vi "Graphe_XY.vi"(0 "Graphe":T1(graph), 3 "Tableau de chaînes":string[](array[string])) -> ()   [LabVIEW 2013]
uses:
  <vilib>/Utility/miscctls.llb/LVPositionTypeDef.ctl
  <vilib>/Utility/miscctls.llb/LVPointTypeDef.ctl
panel:
  in  "Bouton Aide":bool
  in  "Active maths":bool
  out "Nbre courbes":i32
  in  "Quitter graphe":bool
  in  "Palette:Outil actif":i32
  in  "Curseur visible":bool
  in  "Tout sélectionner":bool
  in  "Curseur":u16(ring)
  in  "Quadrillage":u16(ring)=1 items=["Sans", "Horizontal", "Vertical", "Tout"]
  in  "Mini":dbl max=19.999 format="%#.3f"
  in  "Maxi":dbl min=0.001 format="%#.3f"
  in  "Echelle Y":u16(ring) items=["Manu"=0, "Auto"=2]
  out "Y":dbl format="%#.3g"
  out "X":timestamp format="%<%X\n%x>T"
  out "residue 2":dbl caption="résidu"
  out "offset":dbl
  out "damping":dbl caption="atténuation"
  out "amplitude":dbl
  out "R-square":dbl caption="R carré"
  out "residue":dbl caption="résidu"
  out "intercept":dbl caption="interception"
  out "slope":dbl caption="pente"
  out "Intégrale":dbl format="%0.4f"
  out "variance":dbl format="%0.2f"
  out "standard deviation":dbl caption="écart-type" format="%0.2f"
  out "valeur max":dbl
  out "valeur min":dbl
  out "mean":dbl caption="moyenne" format="%0.2f"
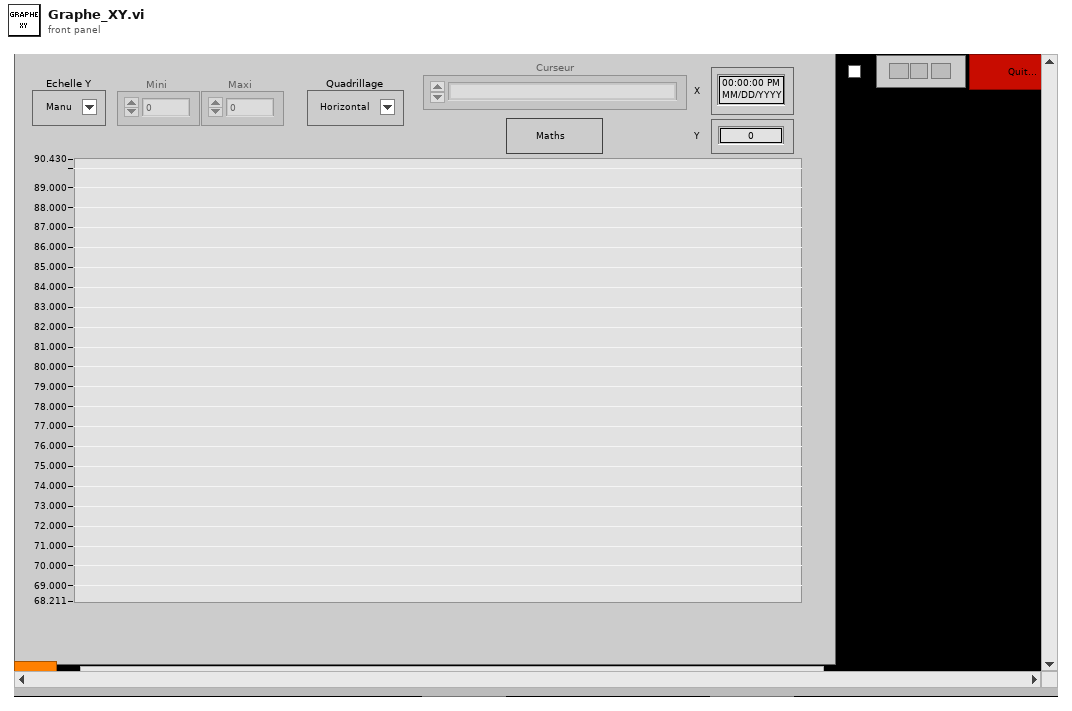
[diagram p1: front panel]
types:
  T1 = cluster{"Horodatage":timestamp[], "Donnees":dbl[]}[]
  T2 = typedef "LVPositionTypeDef.ctl" = cluster{"Left":i32, "Top":i32}
  T3 = typedef "LVPointTypeDef.ctl" = cluster{"Horizontal":i16, "Vertical":i16}
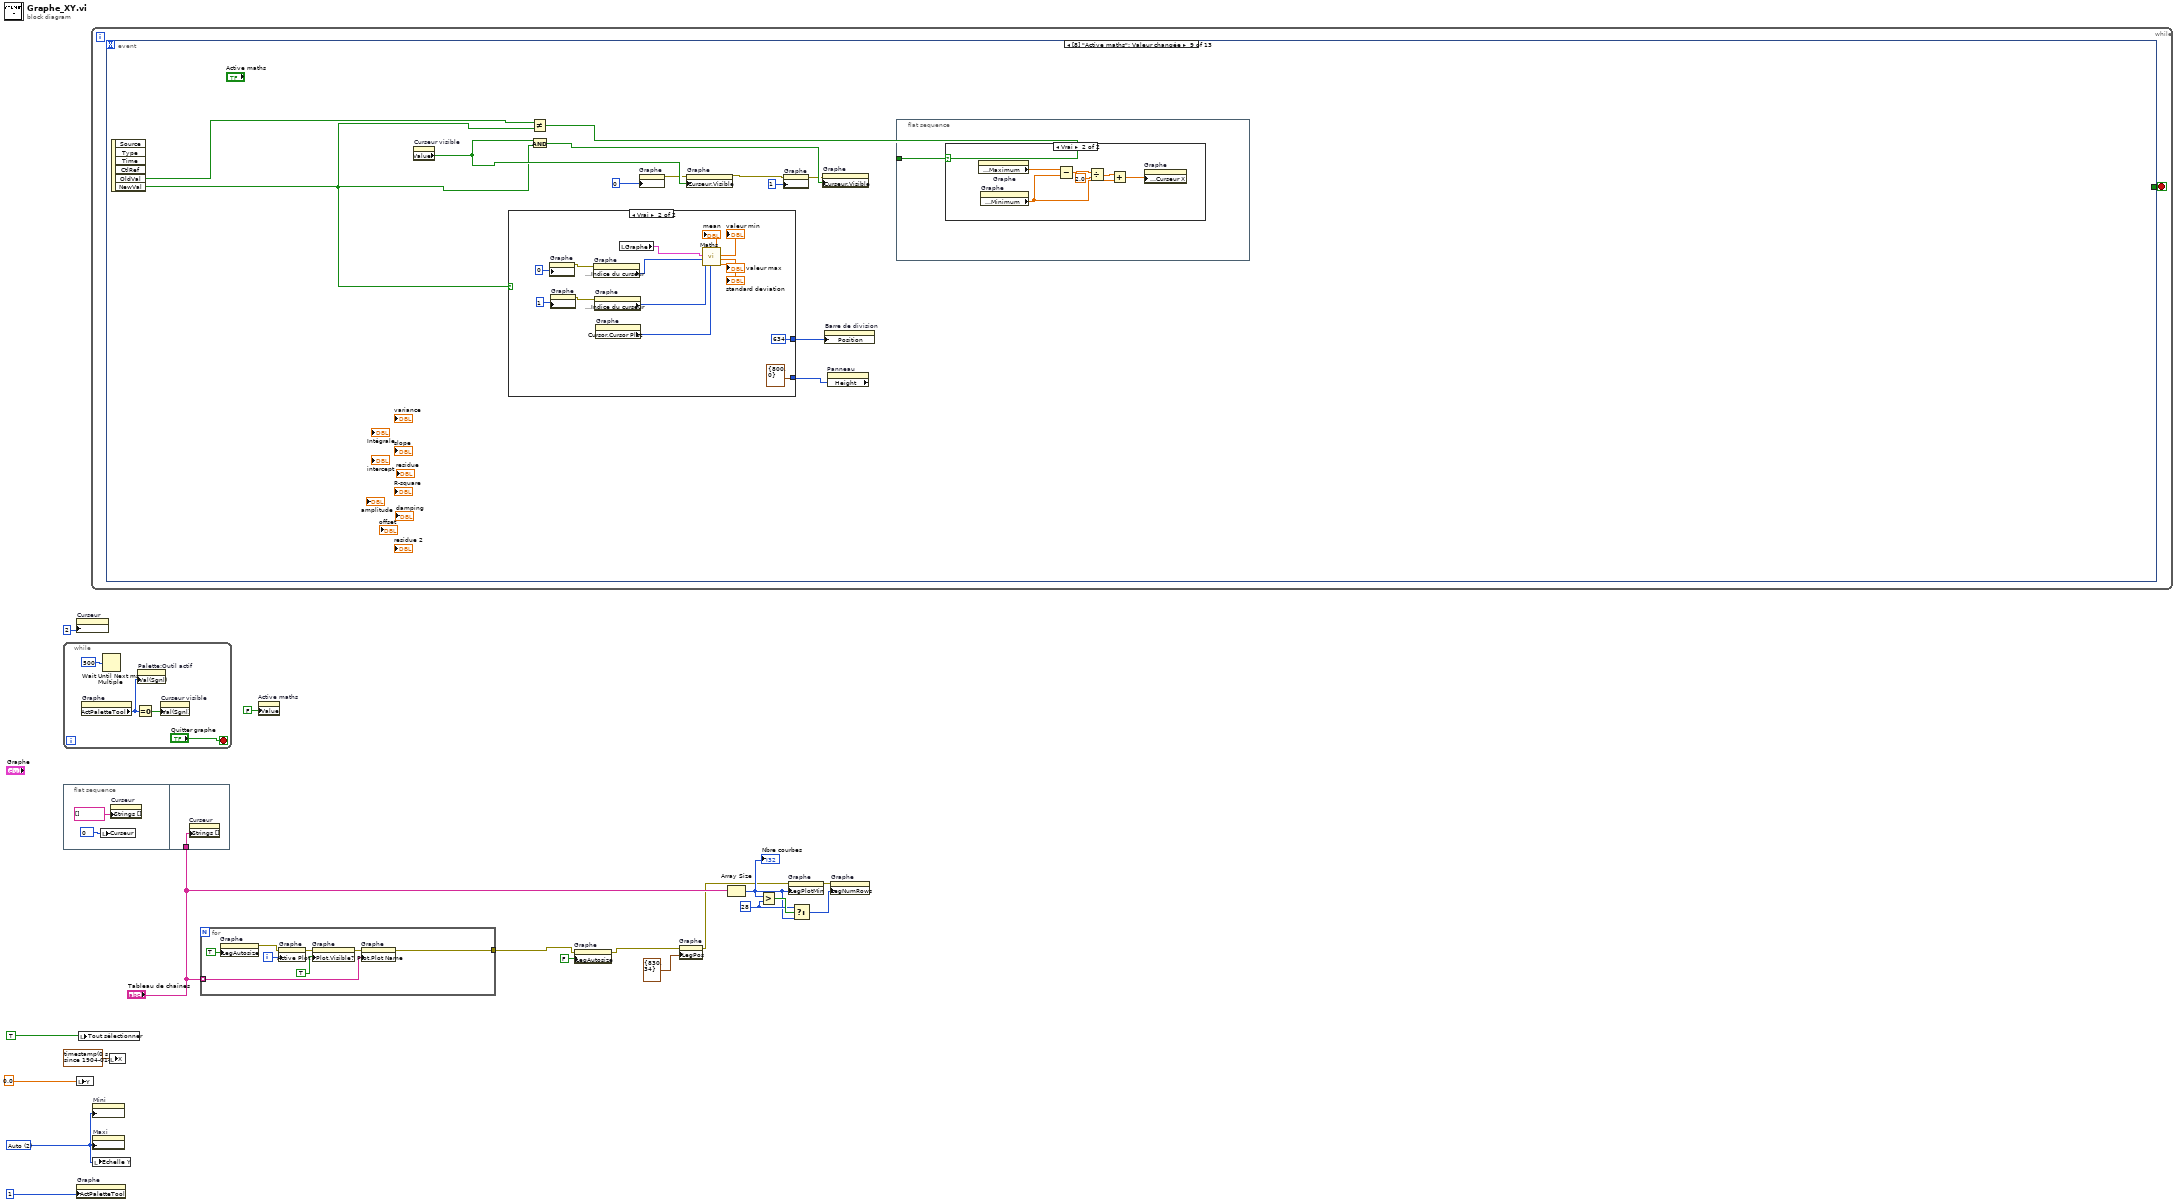
[diagram p0: block diagram]
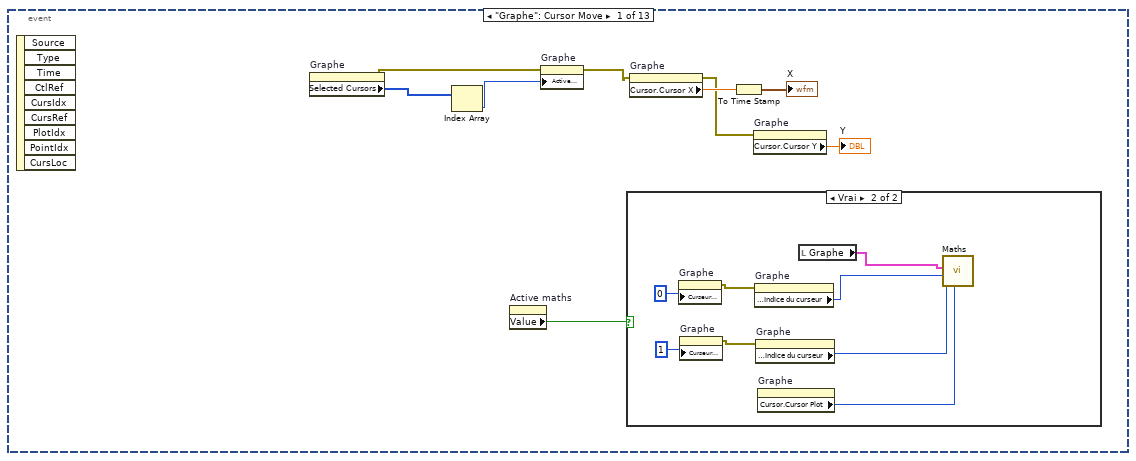
[diagram p2: hidden frame]
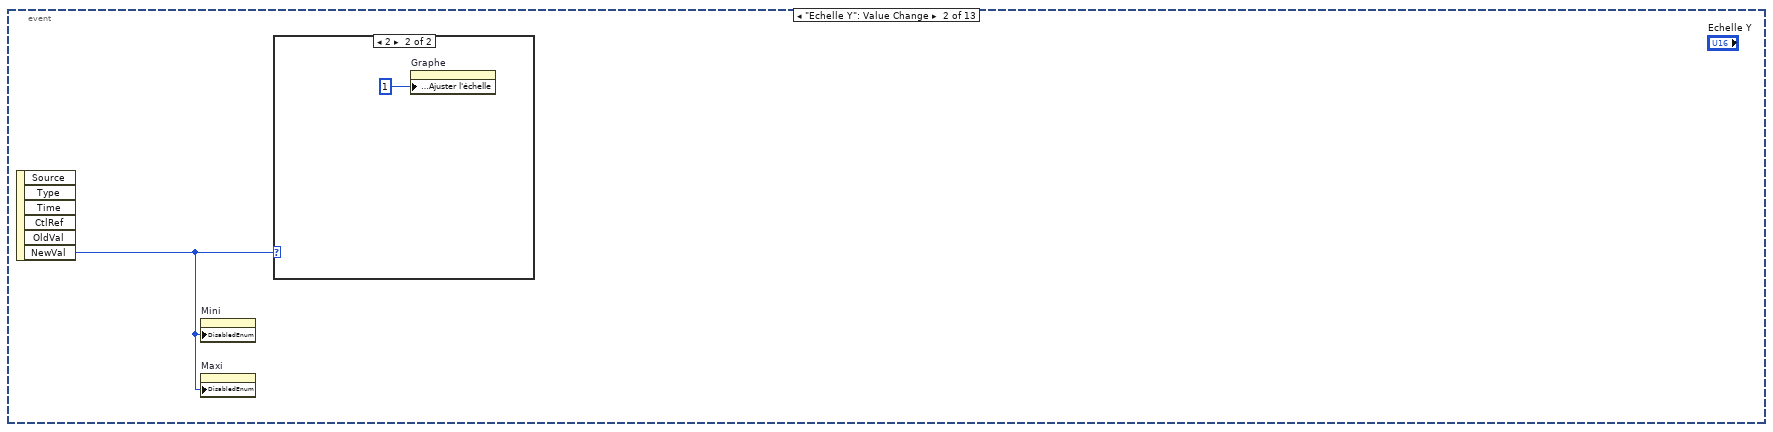
[diagram p4: hidden frame]
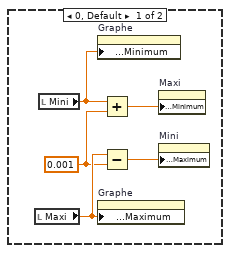
[diagram p5: hidden frame]
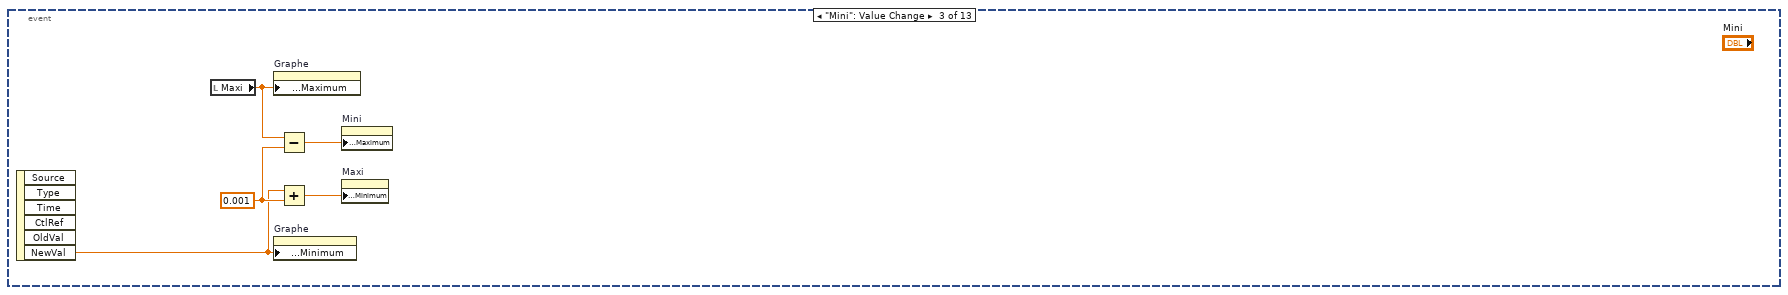
[diagram p6: hidden frame]
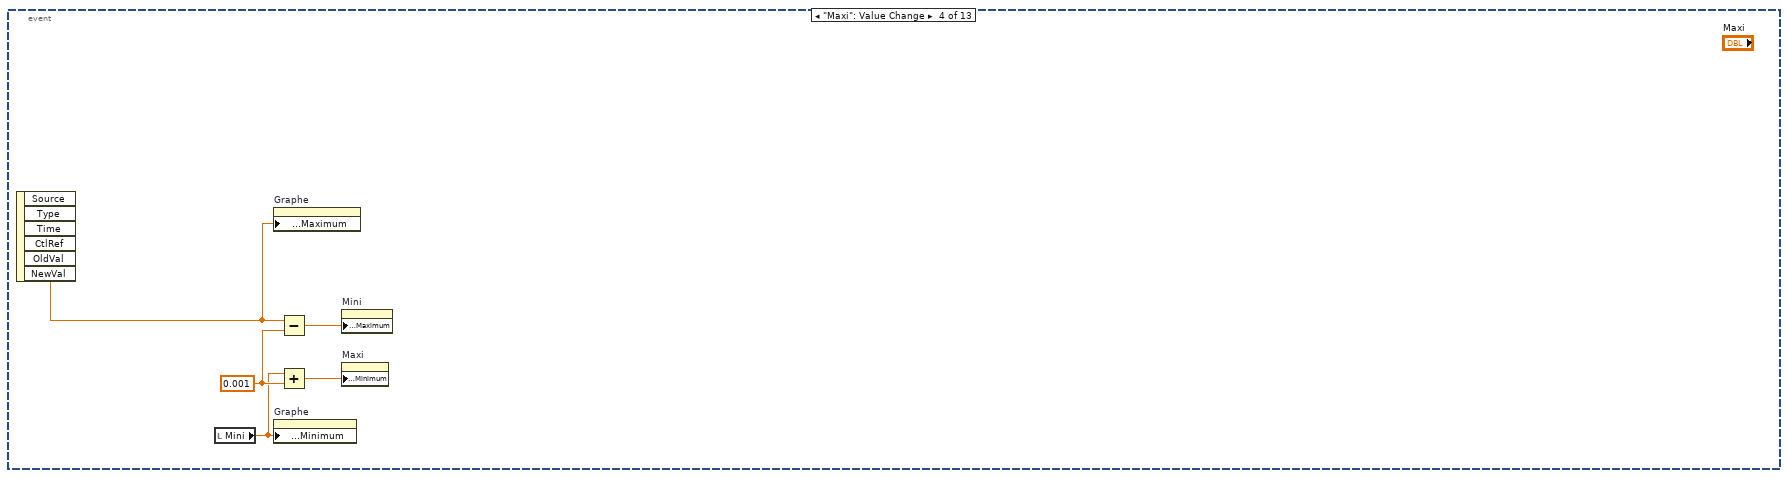
[diagram p7: hidden frame]
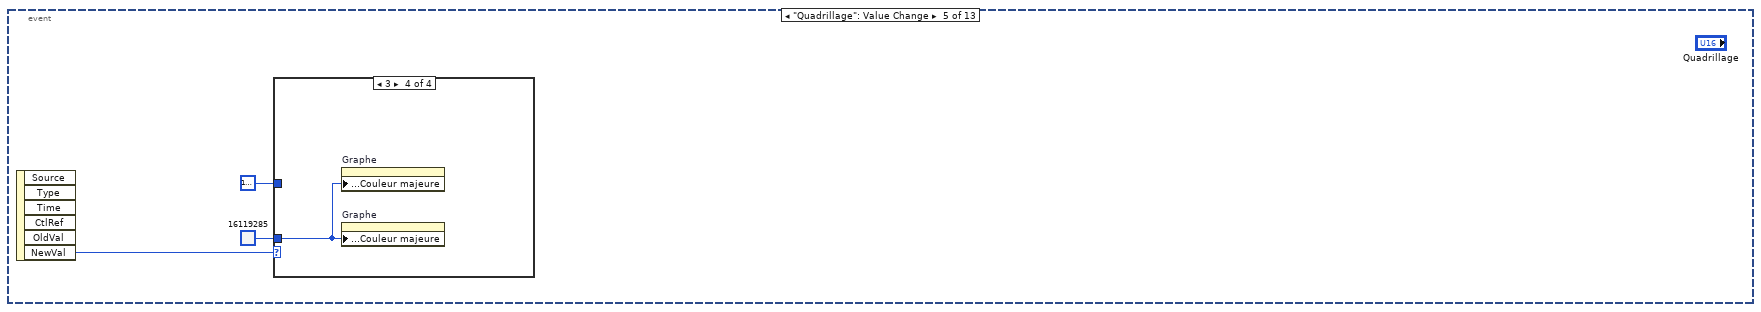
[diagram p8: hidden frame]
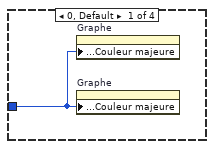
[diagram p9: hidden frame]
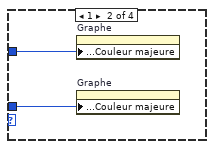
[diagram p10: hidden frame]
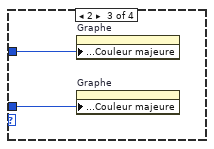
[diagram p11: hidden frame]
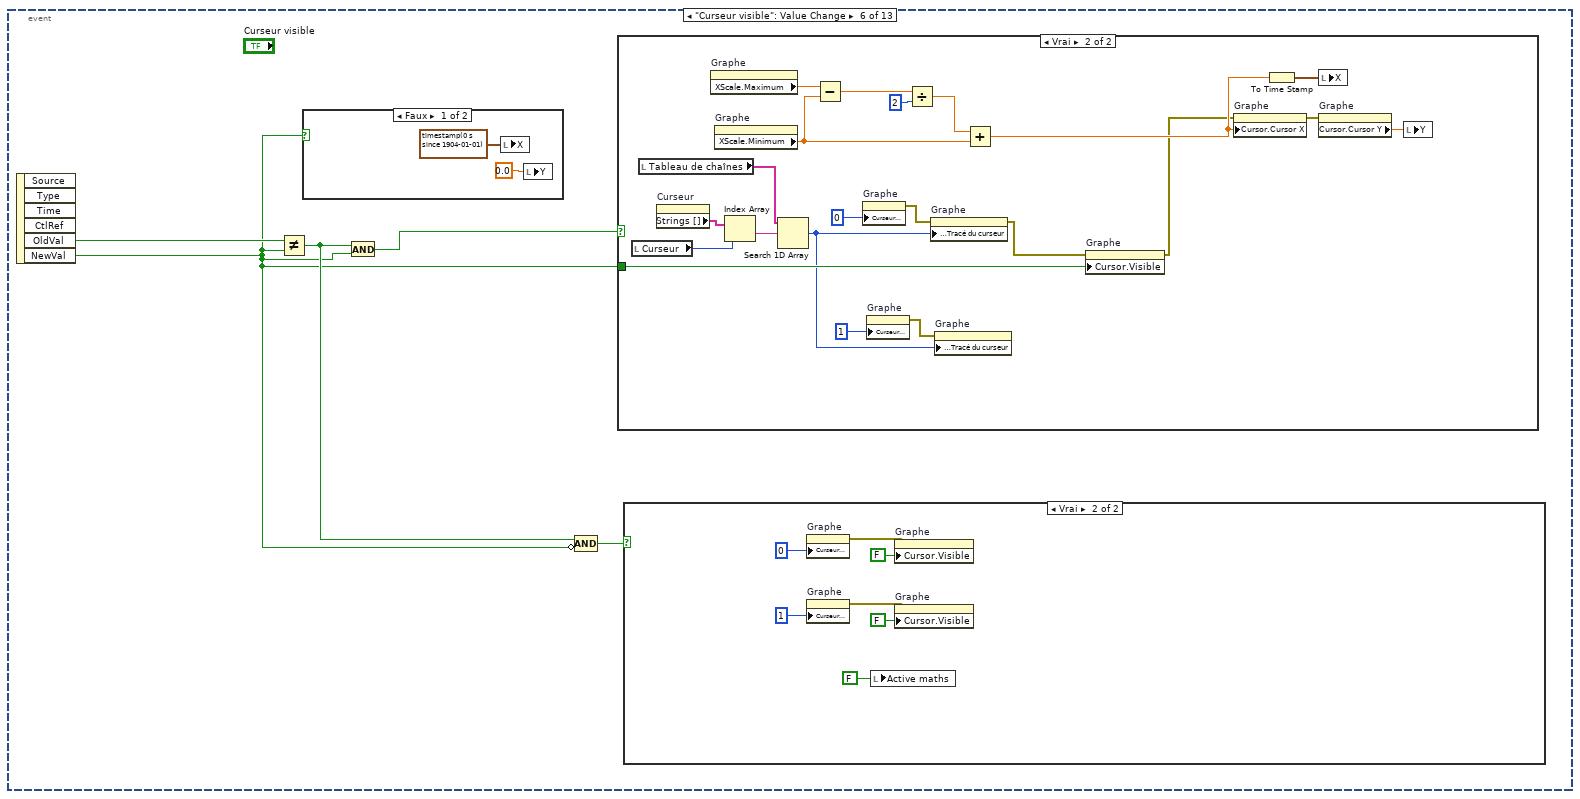
[diagram p12: hidden frame]
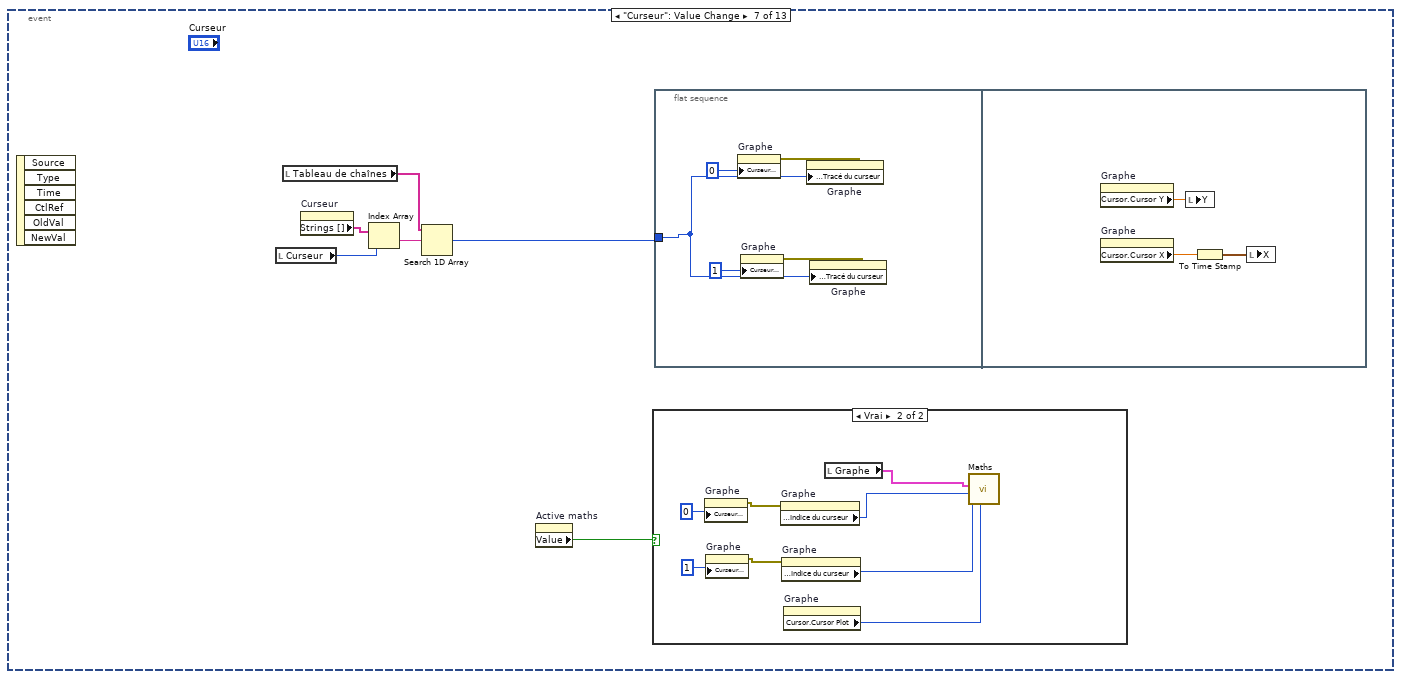
[diagram p16: hidden frame]
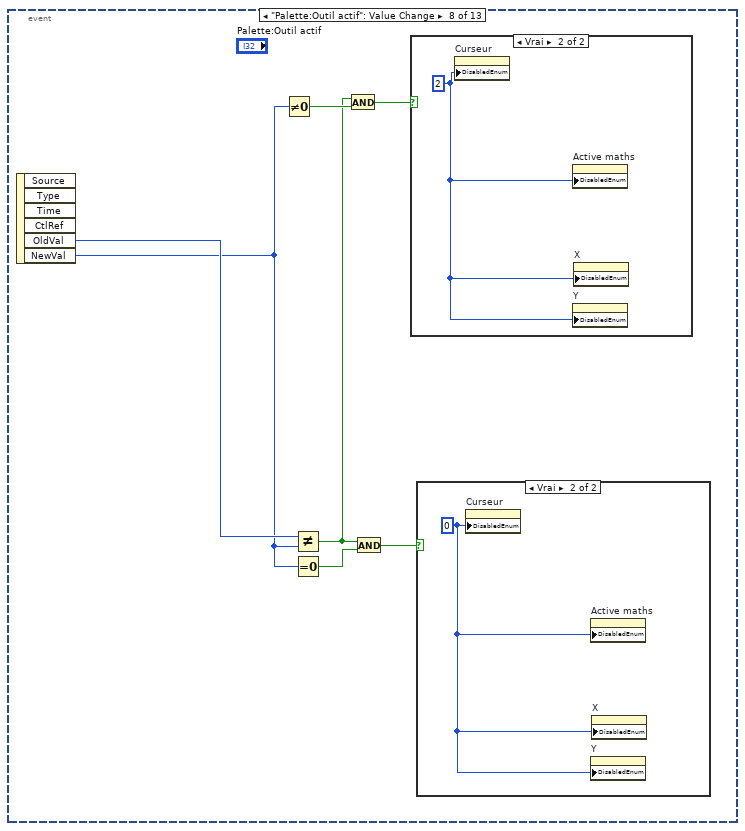
[diagram p18: hidden frame]
diagram:
  w9 = 28 ("y")
  w18 = u16 2 items=["Manu"=0, "Auto"=2] ("Echelle Y")
  n1 = while {
    stop <- "Quitter graphe" stop-if-true
    n2 = property on="Graphe" class="GraphXY (strict)"() -> ("ActPaletteTool"=w20:i32)  [unwired: 2 in, 2 out]
    n3 = Wait Until Next ms Multiple(millisecond multiple=u32 500 ("n millisecondes")) -> ()  [unwired: 1 out]
    n4 = Equal To 0?(x=w20) -> (x = 0?=w21:bool)
    n5 = property on="Palette:Outil actif" class="NumNb (strict)"("Val(Sgnl)"=w20) -> ()  [unwired: 2 in, 2 out]
    n6 = property on="Curseur visible" class="Bool (strict)"("Val(Sgnl)"=w21) -> ()  [unwired: 2 in, 2 out]
  }
  n7 = flat-sequence {
    tunnel: "Tableau de chaînes" -> [w25]
    frame #0 {
      w24 = u16 0 items=[""] ("Curseur")
      n8 = local write "Curseur"(w24) -> ()
      n9 = property on="Curseur" class="MDér (strict)"("Strings []"=string[] [] ("Chaînes []")) -> ()  [unwired: 2 in, 2 out]
    }
    frame #1 {
      n10 = property on="Curseur" class="MDér (strict)"("Strings []"=w25) -> ()  [unwired: 2 in, 2 out]
    }
  }
  n11 = property on="Curseur" class="MDér (strict)"("DisabledEnum"=i8 2 ("cas vrai")) -> ()  [unwired: 2 in, 2 out]
  n12 = local write "Y"(0.0 ("Y")) -> ()
  n13 = property on="Graphe" class="GraphXY (strict)"("ActPaletteTool"=1 ("Palette:Outil actif")) -> ()  [unwired: 2 in, 2 out]
  n14 = local write "Tout sélectionner"(TRUE ("Tout sélectionner")) -> ()
  n15 = while {
    stop <- w26 stop-if-true
    n16 = event shown="[8] \"Active maths\": Valeur changée" {
      selector: _ -> [_ _ _ _ _ _ _ _ _ _ _ _ _]
      dyn-events: _ -> [_ _ _ _ _ _ _ _ _ _ _ _ _]
      timeout: _ -> [_ _ _ _ _ _ _ _ _ _ _ _ _]
      tunnel: [_ _ _ _ _ _ _ _ _ _ _ w241 _] -> w26
      event "Graphe": Cursor Move {
        n17 = event-data() -> ()  [unwired: 1 in, 9 out]
        n18 = property on="Graphe" class="GraphXY (strict)"() -> (error out=w29:errorcluster, "Selected Cursors"=w31:u32[])  [unwired: 2 in, 1 out]
        n19 = Index Array(array=w31) -> (element=w30:u32)  [unwired: 1 in]
        n20 = property on="Active maths" class="Bool (strict)"() -> ("Value"=w27:bool)  [unwired: 2 in, 2 out]
        n21 = property on="Graphe" class="GraphXY (strict)"(error in=w29, "Active Cursor"=w30) -> (error out=w28:errorcluster)  [unwired: 1 in, 1 out]
        n22 = case shown="Vrai" w27 {
          frame False {
          }
          frame True {
            n23 = property on="Graphe" class="GraphXY (strict)"("Curseur actif"=u32 0) -> (error out=w43:errorcluster)  [unwired: 2 in, 1 out]
            n24 = property on="Graphe" class="GraphXY (strict)"("Curseur actif"=u32 1) -> (error out=w39:errorcluster)  [unwired: 2 in, 1 out]
            n25 = property on="Graphe" class="GraphXY (strict)"(error in=w43) -> ("Curseur.Indice du curseur"=w41:i32)  [unwired: 1 in, 2 out]
            n26 = property on="Graphe" class="GraphXY (strict)"(error in=w39) -> ("Curseur.Indice du curseur"=w38:i32)  [unwired: 1 in, 2 out]
            n27 = property on="Graphe" class="GraphXY (strict)"() -> ("Cursor.Cursor Plot"=w37:i32)  [unwired: 2 in, 2 out]
            n28 = local read "Graphe"() -> (w36:T1)
            n29 = call "Maths.vi"("Curseur tracé"=w37, "Indice curseur 2"=w38, "Indice curseur 1"=w41, "Graphe"=w36) -> ()  [unwired: 4 in, 4 out]
          }
        }
        n30 = property on="Graphe" class="GraphXY (strict)"(error in=w28) -> (error out=w32:errorcluster, "Cursor.Cursor X"=w34:dbl)  [unwired: 1 in, 1 out]
        n31 = To Time Stamp(1:w34) -> (0:→"X":timestamp)
        n32 = property on="Graphe" class="GraphXY (strict)"(error in=w32) -> ("Cursor.Cursor Y"=→"Y":dbl)  [unwired: 1 in, 2 out]
      }
      event "Echelle Y": Value Change {
        n33 = event-data() -> ("NewVal"=w44:u16)  [unwired: 1 in, 5 out]
        n34 = property on="Mini" class="NumNb (strict)"("DisabledEnum"=w44) -> ()  [unwired: 2 in, 2 out]
        n35 = property on="Maxi" class="NumNb (strict)"("DisabledEnum"=w44) -> ()  [unwired: 2 in, 2 out]
        n36 = case shown="2" w44 {
          frame 0, Default {
            w48 = 0.001 ("y")
            n37 = local read "Maxi"() -> (w49:dbl)
            n38 = local read "Mini"() -> (w45:dbl)
            n39 = property on="Graphe" class="GraphXY (strict)"("Échelle des Y.Gamme:Minimum"=w45) -> ()  [unwired: 2 in, 2 out]
            n40 = property on="Graphe" class="GraphXY (strict)"("Échelle des Y.Gamme:Maximum"=w49) -> ()  [unwired: 2 in, 2 out]
            n41 = Add(x=w45, y=w48) -> (x+y=w46:dbl)
            n42 = Subtract(x=w49, y=w48) -> (x-y=w47:dbl)
            n43 = property on="Maxi" class="NumNb (strict)"("Limites d'entrée des données:Minimum"=w46) -> ()  [unwired: 2 in, 2 out]
            n44 = property on="Mini" class="NumNb (strict)"("Limites d'entrée des données:Maximum"=w47) -> ()  [unwired: 2 in, 2 out]
          }
          frame 2 {
            n45 = property on="Graphe" class="GraphXY (strict)"("Échelle des Y.Ajuster l'échelle"=u8 1 ("Échelle Y.Ajuster l'échelle")) -> ()  [unwired: 2 in, 2 out]
          }
        }
      }
      event "Mini": Value Change {
        w54 = 0.001 ("y")
        n46 = event-data() -> ("NewVal"=w51:dbl)  [unwired: 1 in, 5 out]
        n47 = local read "Maxi"() -> (w55:dbl)
        n48 = property on="Graphe" class="GraphXY (strict)"("Échelle des Y.Gamme:Maximum"=w55) -> ()  [unwired: 2 in, 2 out]
        n49 = property on="Graphe" class="GraphXY (strict)"("Échelle des Y.Gamme:Minimum"=w51) -> ()  [unwired: 2 in, 2 out]
        n50 = Subtract(x=w55, y=w54) -> (x-y=w53:dbl)
        n51 = Add(x=w51, y=w54) -> (x+y=w52:dbl)
        n52 = property on="Mini" class="NumNb (strict)"("Limites d'entrée des données:Maximum"=w53) -> ()  [unwired: 2 in, 2 out]
        n53 = property on="Maxi" class="NumNb (strict)"("Limites d'entrée des données:Minimum"=w52) -> ()  [unwired: 2 in, 2 out]
      }
      event "Maxi": Value Change {
        w60 = 0.001 ("y")
        n54 = event-data() -> ("NewVal"=w57:dbl)  [unwired: 1 in, 5 out]
        n55 = local read "Mini"() -> (w56:dbl)
        n56 = property on="Graphe" class="GraphXY (strict)"("Échelle des Y.Gamme:Maximum"=w57) -> ()  [unwired: 2 in, 2 out]
        n57 = property on="Graphe" class="GraphXY (strict)"("Échelle des Y.Gamme:Minimum"=w56) -> ()  [unwired: 2 in, 2 out]
        n58 = Subtract(x=w57, y=w60) -> (x-y=w59:dbl)
        n59 = Add(x=w56, y=w60) -> (x+y=w58:dbl)
        n60 = property on="Mini" class="NumNb (strict)"("Limites d'entrée des données:Maximum"=w59) -> ()  [unwired: 2 in, 2 out]
        n61 = property on="Maxi" class="NumNb (strict)"("Limites d'entrée des données:Minimum"=w58) -> ()  [unwired: 2 in, 2 out]
      }
      event "Quadrillage": Value Change {
        n62 = event-data() -> ("NewVal"=w63:u16)  [unwired: 1 in, 5 out]
        n63 = case shown="3" w63 {
          tunnel: u32 16119285 -> [_ w66 w68 w69]
          tunnel: u32 16777216 -> [w64 w65 w67 _]
          frame 0, Default {
            n64 = property on="Graphe" class="GraphXY (strict)"("Échelle des X.Couleurs de grille:Couleur majeure"=w64) -> ()  [unwired: 2 in, 2 out]
            n65 = property on="Graphe" class="GraphXY (strict)"("Échelle des Y.Couleurs de grille:Couleur majeure"=w64) -> ()  [unwired: 2 in, 2 out]
          }
          frame 1 {
            n66 = property on="Graphe" class="GraphXY (strict)"("Échelle des X.Couleurs de grille:Couleur majeure"=w65) -> ()  [unwired: 2 in, 2 out]
            n67 = property on="Graphe" class="GraphXY (strict)"("Échelle des Y.Couleurs de grille:Couleur majeure"=w66) -> ()  [unwired: 2 in, 2 out]
          }
          frame 2 {
            n68 = property on="Graphe" class="GraphXY (strict)"("Échelle des Y.Couleurs de grille:Couleur majeure"=w67) -> ()  [unwired: 2 in, 2 out]
            n69 = property on="Graphe" class="GraphXY (strict)"("Échelle des X.Couleurs de grille:Couleur majeure"=w68) -> ()  [unwired: 2 in, 2 out]
          }
          frame 3 {
            n70 = property on="Graphe" class="GraphXY (strict)"("Échelle des X.Couleurs de grille:Couleur majeure"=w69) -> ()  [unwired: 2 in, 2 out]
            n71 = property on="Graphe" class="GraphXY (strict)"("Échelle des Y.Couleurs de grille:Couleur majeure"=w69) -> ()  [unwired: 2 in, 2 out]
          }
        }
      }
      event "Curseur visible": Value Change {
        n72 = event-data() -> ("OldVal"=w74:bool, "NewVal"=w70:bool)  [unwired: 1 in, 4 out]
        n73 = Not Equal?(x=w74, y=w70) -> (x != y?=w72:bool)
        n74 = case shown="Faux" w70 {
          frame False {
            n75 = local write "X"(timestamp(0 s since 1904-01-01) ("X")) -> ()
            n76 = local write "Y"(0.0 ("Y")) -> ()
          }
          frame True {
          }
        }
        n77 = And(x=w72, y=w70) -> (x .and. y?=w73:bool)
        n78 = Compound Arithmetic op=AND(w72, invert w70) -> (w71:bool)
        n79 = case shown="Vrai" w73 {
          tunnel: w70 -> [_ w94]
          frame False {
          }
          frame True {
            n80 = local read "Curseur"() -> (w89:u16)
            n81 = local read "Tableau de chaînes"() -> (w92:string[])
            n82 = property on="Curseur" class="MDér (strict)"() -> ("Strings []"=w90:string[])  [unwired: 2 in, 2 out]
            n83 = property on="Graphe" class="GraphXY (strict)"() -> ("XScale.Maximum"=w103:dbl)  [unwired: 2 in, 2 out]
            n84 = property on="Graphe" class="GraphXY (strict)"() -> ("XScale.Minimum"=w100:dbl)  [unwired: 2 in, 2 out]
            n85 = Index Array(array=w90, index=w89) -> (element=w91:string)
            n86 = Search 1D Array(1D array=w92, element=w91) -> (index of element=w86:i32)  [unwired: 1 in]
            n87 = Subtract(x=w103, y=w100) -> (x-y=w102:dbl)
            n88 = property on="Graphe" class="GraphXY (strict)"("Curseur actif"=u32 0) -> (error out=w93:errorcluster)  [unwired: 2 in, 1 out]
            n89 = property on="Graphe" class="GraphXY (strict)"("Curseur actif"=u32 1) -> (error out=w88:errorcluster)  [unwired: 2 in, 1 out]
            n90 = Divide(x=w102, y=2) -> (x/y=w101:dbl)
            n91 = property on="Graphe" class="GraphXY (strict)"(error in=w93, "Curseur.Tracé du curseur"=w86) -> (error out=w84:errorcluster)  [unwired: 1 in, 1 out]
            n92 = property on="Graphe" class="GraphXY (strict)"(error in=w88, "Curseur.Tracé du curseur"=w86) -> ()  [unwired: 1 in, 2 out]
            n93 = Add(x=w101, y=w100) -> (x+y=w97:dbl)
            n94 = property on="Graphe" class="GraphXY (strict)"(error in=w84, "Cursor.Visible"=w94) -> (error out=w85:errorcluster)  [unwired: 1 in, 1 out]
            n95 = property on="Graphe" class="GraphXY (strict)"(error in=w85, "Cursor.Cursor X"=w97) -> (error out=w96:errorcluster)  [unwired: 1 in, 1 out]
            n96 = To Time Stamp(1:w97) -> (0:w98:timestamp)
            n97 = local write "X"(w98) -> ()
            n98 = property on="Graphe" class="GraphXY (strict)"(error in=w96) -> ("Cursor.Cursor Y"=w99:dbl)  [unwired: 1 in, 2 out]
            n99 = local write "Y"(w99) -> ()
          }
        }
        n100 = case shown="Vrai" w71 {
          frame False {
          }
          frame True {
            n101 = property on="Graphe" class="GraphXY (strict)"("Curseur actif"=u32 0) -> (error out=w80:errorcluster)  [unwired: 2 in, 1 out]
            n102 = property on="Graphe" class="GraphXY (strict)"("Curseur actif"=u32 1) -> (error out=w77:errorcluster)  [unwired: 2 in, 1 out]
            n103 = local write "Active maths"(FALSE ("Selection math")) -> ()
            n104 = property on="Graphe" class="GraphXY (strict)"(error in=w80, "Cursor.Visible"=FALSE ("Curseur.Visible")) -> ()  [unwired: 1 in, 2 out]
            n105 = property on="Graphe" class="GraphXY (strict)"(error in=w77, "Cursor.Visible"=FALSE ("Curseur.Visible")) -> ()  [unwired: 1 in, 2 out]
          }
        }
      }
      event "Curseur": Value Change {
        n106 = event-data() -> ()  [unwired: 1 in, 6 out]
        n107 = local read "Curseur"() -> (w106:u16)
        n108 = local read "Tableau de chaînes"() -> (w109:string[])
        n109 = property on="Curseur" class="MDér (strict)"() -> ("Strings []"=w107:string[])  [unwired: 2 in, 2 out]
        n110 = Index Array(array=w107, index=w106) -> (element=w108:string)
        n111 = Search 1D Array(1D array=w109, element=w108) -> (index of element=w105:i32)  [unwired: 1 in]
        n112 = property on="Active maths" class="Bool (strict)"() -> ("Value"=w110:bool)  [unwired: 2 in, 2 out]
        n113 = case shown="Vrai" w110 {
          frame False {
          }
          frame True {
            n114 = property on="Graphe" class="GraphXY (strict)"("Curseur actif"=u32 0) -> (error out=w118:errorcluster)  [unwired: 2 in, 1 out]
            n115 = property on="Graphe" class="GraphXY (strict)"("Curseur actif"=u32 1) -> (error out=w114:errorcluster)  [unwired: 2 in, 1 out]
            n116 = property on="Graphe" class="GraphXY (strict)"(error in=w118) -> ("Curseur.Indice du curseur"=w116:i32)  [unwired: 1 in, 2 out]
            n117 = property on="Graphe" class="GraphXY (strict)"(error in=w114) -> ("Curseur.Indice du curseur"=w113:i32)  [unwired: 1 in, 2 out]
            n118 = property on="Graphe" class="GraphXY (strict)"() -> ("Cursor.Cursor Plot"=w112:i32)  [unwired: 2 in, 2 out]
            n119 = local read "Graphe"() -> (w111:T1)
            n120 = call "Maths.vi"("Curseur tracé"=w112, "Indice curseur 2"=w113, "Indice curseur 1"=w116, "Graphe"=w111) -> ()  [unwired: 4 in, 4 out]
          }
        }
        n121 = flat-sequence {
          tunnel: w105 -> [w119]
          frame #0 {
            n122 = property on="Graphe" class="GraphXY (strict)"("Curseur actif"=u32 0) -> (error out=w122:errorcluster)  [unwired: 2 in, 1 out]
            n123 = property on="Graphe" class="GraphXY (strict)"("Curseur actif"=u32 1) -> (error out=w121:errorcluster)  [unwired: 2 in, 1 out]
            n124 = property on="Graphe" class="GraphXY (strict)"(error in=w122, "Curseur.Tracé du curseur"=w119) -> ()  [unwired: 1 in, 2 out]
            n125 = property on="Graphe" class="GraphXY (strict)"(error in=w121, "Curseur.Tracé du curseur"=w119) -> ()  [unwired: 1 in, 2 out]
          }
          frame #1 {
            n126 = property on="Graphe" class="GraphXY (strict)"() -> ("Cursor.Cursor Y"=w126:dbl)  [unwired: 2 in, 2 out]
            n127 = property on="Graphe" class="GraphXY (strict)"() -> ("Cursor.Cursor X"=w124:dbl)  [unwired: 2 in, 2 out]
            n128 = local write "Y"(w126) -> ()
            n129 = To Time Stamp(1:w124) -> (0:w125:timestamp)
            n130 = local write "X"(w125) -> ()
          }
        }
      }
      event "Palette:Outil actif": Value Change {
        n131 = event-data() -> ("OldVal"=w133:i32, "NewVal"=w129:i32)  [unwired: 1 in, 4 out]
        n132 = Not Equal To 0?(x=w129) -> (x != 0?=w130:bool)
        n133 = Not Equal?(x=w133, y=w129) -> (x != y?=w128:bool)
        n134 = Equal To 0?(x=w129) -> (x = 0?=w127:bool)
        n135 = And(x=w128, y=w130) -> (x .and. y?=w131:bool)
        n136 = And(x=w128, y=w127) -> (x .and. y?=w132:bool)
        n137 = case shown="Vrai" w131 {
          frame False {
          }
          frame True {
            w134 = i8 2 ("cas vrai")
            n138 = property on="Curseur" class="MDér (strict)"("DisabledEnum"=w134) -> ()  [unwired: 2 in, 2 out]
            n139 = property on="Active maths" class="Bool (strict)"("DisabledEnum"=w134) -> ()  [unwired: 2 in, 2 out]
            n140 = property on="Y" class="NumNb (strict)"("DisabledEnum"=w134) -> ()  [unwired: 2 in, 2 out]
            n141 = property on="X" class="TempsAbs (strict)"("DisabledEnum"=w134) -> ()  [unwired: 2 in, 2 out]
          }
        }
        n142 = case shown="Vrai" w132 {
          frame False {
          }
          frame True {
            w135 = i8 0 ("cas vrai")
            n143 = property on="Curseur" class="MDér (strict)"("DisabledEnum"=w135) -> ()  [unwired: 2 in, 2 out]
            n144 = property on="Active maths" class="Bool (strict)"("DisabledEnum"=w135) -> ()  [unwired: 2 in, 2 out]
            n145 = property on="Y" class="NumNb (strict)"("DisabledEnum"=w135) -> ()  [unwired: 2 in, 2 out]
            n146 = property on="X" class="TempsAbs (strict)"("DisabledEnum"=w135) -> ()  [unwired: 2 in, 2 out]
          }
        }
      }
      event "Active maths": Value Change {
        n147 = event-data() -> ("OldVal"=w145:bool, "NewVal"=w138:bool)  [unwired: 1 in, 4 out]
        n148 = property on="Curseur visible" class="Bool (strict)"() -> ("Value"=w143:bool)  [unwired: 2 in, 2 out]
        n149 = Not Equal?(x=w145, y=w138) -> (x != y?=w147:bool)
        n150 = And(x=w143, y=w138) -> (x .and. y?=w146:bool)
        n151 = property on="Graphe" class="GraphXY (strict)"("Curseur actif"=u32 0) -> (error out=w140:errorcluster)  [unwired: 2 in, 1 out]
        n152 = property on="Graphe" class="GraphXY (strict)"(error in=w140, "Curseur.Visible"=w143) -> (error out=w142:errorcluster)  [unwired: 1 in, 1 out]
        n153 = property on="Graphe" class="GraphXY (strict)"(error in=w142, "Curseur actif"=u32 1) -> (error out=w139:errorcluster)  [unwired: 1 in, 1 out]
        n154 = property on="Graphe" class="GraphXY (strict)"(error in=w139, "Curseur.Visible"=w146) -> ()  [unwired: 1 in, 2 out]
        n155 = property on="Panneau" class="Pann"() -> ("Height"=w137:u32)  [unwired: 2 in, 2 out]
        n156 = case shown="Vrai" w138 {
          tunnel: [634 ("Position de la barre de division") 634 ("Position de la barre de division")] -> w136
          tunnel: w137 -> [T3 {"Horizontal"=636, "Vertical"=0} ("Taille minimale de panneau") T3 {"Horizontal"=800, "Vertical"=0} ("Taille minimale de panneau")]
          frame False {
          }
          frame True {
            n157 = property on="Graphe" class="GraphXY (strict)"("Curseur actif"=u32 0) -> (error out=w163:errorcluster)  [unwired: 2 in, 1 out]
            n158 = property on="Graphe" class="GraphXY (strict)"("Curseur actif"=u32 1) -> (error out=w159:errorcluster)  [unwired: 2 in, 1 out]
            n159 = property on="Graphe" class="GraphXY (strict)"(error in=w163) -> ("Curseur.Indice du curseur"=w161:i32)  [unwired: 1 in, 2 out]
            n160 = property on="Graphe" class="GraphXY (strict)"(error in=w159) -> ("Curseur.Indice du curseur"=w158:i32)  [unwired: 1 in, 2 out]
            n161 = property on="Graphe" class="GraphXY (strict)"() -> ("Cursor.Cursor Plot"=w157:i32)  [unwired: 2 in, 2 out]
            n162 = local read "Graphe"() -> (w156:T1)
            n163 = call "Maths.vi"("Curseur tracé"=w157, "Indice curseur 2"=w158, "Indice curseur 1"=w161, "Graphe"=w156) -> ("standard deviation"=→"standard deviation":dbl, "valeur max"=→"valeur max":dbl, "valeur min"=→"valeur min":dbl, "mean"=→"mean":dbl)  [unwired: 4 in]
          }
        }
        n164 = property on="Barre de division" class="BarreDiv"("Position"=w136) -> ()  [unwired: 2 in, 2 out]
        n165 = flat-sequence {
          tunnel: w147 -> [w164]
          frame #0 {
            n166 = case shown="Vrai" w164 {
              frame False {
              }
              frame True {
                n167 = property on="Graphe" class="GraphXY (strict)"() -> ("Échelle des X.Gamme:Maximum"=w167:dbl)  [unwired: 2 in, 2 out]
                n168 = property on="Graphe" class="GraphXY (strict)"() -> ("Échelle des X.Gamme:Minimum"=w169:dbl)  [unwired: 2 in, 2 out]
                n169 = Subtract(x=w167, y=w169) -> (x-y=w166:dbl)
                n170 = Divide(x=w166, y=2.0) -> (x/y=w168:dbl)
                n171 = Add(x=w168, y=w169) -> (x+y=w170:dbl)
                n172 = property on="Graphe" class="GraphXY (strict)"("Curseur.Position du curseur:Curseur X"=w170) -> ()  [unwired: 2 in, 2 out]
              }
            }
          }
        }
      }
      event "Graphe": Plot Attribute Change {
        n173 = event-data() -> ()  [unwired: 1 in, 8 out]
        n174 = local read "Nbre courbes"() -> (w179:i32)
        n175 = property on="Graphe" class="GraphXY (strict)"() -> ("ActPaletteTool"=w180:i32)  [unwired: 2 in, 2 out]
        n176 = property on="Curseur" class="MDér (strict)"("Strings []"=string[] [] ("Chaînes []")) -> ()  [unwired: 2 in, 2 out]
        n177 = local read "Echelle Y"() -> (w172:u16)
        n178 = Greater?(x=w180, y=u8 1) -> (0:w175:bool)
        n179 = for {
          N: w179 -> [_]
          shift-right: [w209] -> w178
          shift-left: TRUE -> [w208]
          i -> [w206]
          n180 = local read "Tableau de chaînes"() -> (w207:string[])
          n181 = property on="Graphe" class="GraphXY (strict)"("Active Plot"=w206) -> (error out=w210:errorcluster)  [unwired: 2 in, 1 out]
          n182 = property on="Graphe" class="GraphXY (strict)"(error in=w210) -> ("Plot.Visible?"=w204:bool)  [unwired: 1 in, 2 out]
          n183 = Index Array(array=w207, index=w206) -> (element=w205:string)
          n184 = case shown="Vrai" w204 {
            tunnel: w205 -> [_ w213]
            frame False {
            }
            frame True {
              n185 = property on="Curseur" class="MDér (strict)"() -> ("Strings []"=w211:string[])  [unwired: 2 in, 2 out]
              n186 = Array Size(array=w211) -> (size(s)=w212:i32)
              n187 = Insert Into Array(array=w211, index=w212, new element=w213) -> (w214:string[])
              n188 = property on="Curseur" class="MDér (strict)"("Strings []"=w214) -> ()  [unwired: 2 in, 2 out]
            }
          }
          n189 = And(x=w204, y=w208) -> (x .and. y?=w209:bool)
        }
        n190 = Select(t=i8 0 ("cas vrai"), s=w175, f=w172) -> (s? t:f=w176:u16)
        n191 = Select(t=i8 0 ("cas vrai"), s=w175, f=i8 2 ("cas faux")) -> (s? t:f=w182:i8)
        n192 = property on="Graphe" class="GraphXY (strict)"("YScale.ScaleFit"=w176) -> ()  [unwired: 2 in, 2 out]
        n193 = property on="Graphe" class="GraphXY (strict)"("XScale.ScaleFit"=w182) -> ()  [unwired: 2 in, 2 out]
        n194 = flat-sequence {
          tunnel: w178 -> [w184]
          frame #0 {
            n195 = local write "Tout sélectionner"(w184) -> ()
          }
          frame #1 {
            n196 = property on="Curseur" class="MDér (strict)"() -> ("Strings []"=w187:string[])  [unwired: 2 in, 2 out]
            n197 = Index Array(array=w187) -> (element=w188:string)  [unwired: 1 in]
            n198 = Empty String/Path?(string/path=w188) -> (empty?=w186:bool)
            n199 = case shown="Faux" w186 {
              tunnel: w187 -> [w189 w193]
              tunnel: [w189 w190] -> w185
              frame False {
              }
              frame True {
                n200 = Delete From Array(array=w193, length=1 ("longueur"), index=0 ("indice")) -> (array with subset deleted=w190:string[])  [unwired: 1 out]
              }
            }
            n201 = property on="Curseur" class="MDér (strict)"("Strings []"=w185) -> ()  [unwired: 2 in, 2 out]
          }
          frame #2 {
            n202 = local read "Curseur"() -> (w196:u16)
            n203 = local read "Tableau de chaînes"() -> (w199:string[])
            n204 = property on="Curseur" class="MDér (strict)"() -> ("Strings []"=w197:string[])  [unwired: 2 in, 2 out]
            n205 = Index Array(array=w197, index=w196) -> (element=w198:string)
            n206 = Search 1D Array(1D array=w199, element=w198) -> (index of element=w195:i32)  [unwired: 1 in]
            n207 = property on="Graphe" class="GraphXY (strict)"("Curseur actif"=u32 0) -> (error out=w194:errorcluster)  [unwired: 2 in, 1 out]
            n208 = property on="Graphe" class="GraphXY (strict)"(error in=w194, "Curseur.Tracé du curseur"=w195) -> ()  [unwired: 1 in, 2 out]
          }
          frame #3 {
            n209 = property on="Graphe" class="GraphXY (strict)"() -> ("Cursor.Cursor Y"=w201:dbl)  [unwired: 2 in, 2 out]
            n210 = property on="Graphe" class="GraphXY (strict)"() -> ("Cursor.Cursor X"=w203:dbl)  [unwired: 2 in, 2 out]
            n211 = local write "Y"(w201) -> ()
            n212 = To Time Stamp(1:w203) -> (0:w202:timestamp)
            n213 = local write "X"(w202) -> ()
          }
        }
      }
      event "Tout sélectionner": Value Change {
        n214 = event-data() -> ("NewVal"=w228:bool)  [unwired: 1 in, 5 out]
        n215 = flat-sequence {
          frame #0 {
            n216 = local read "Nbre courbes"() -> (w230:i32)
            n217 = for {
              N: w230 -> [_]
              i -> [w232]
              n218 = property on="Graphe" class="GraphXY (strict)"("Active Plot"=w232) -> (error out=w233:errorcluster)  [unwired: 2 in, 1 out]
              n219 = property on="Graphe" class="GraphXY (strict)"(error in=w233, "Plot.Visible?"="Tout sélectionner") -> ()  [unwired: 1 in, 2 out]
            }
          }
          frame #1 {
            n220 = property on="Graphe" class="GraphXY (strict)"() -> ("ActPaletteTool"=w234:i32)  [unwired: 2 in, 2 out]
            n221 = local read "Echelle Y"() -> (w240:u16)
            n222 = property on="Graphe" class="GraphXY (strict)"("YScale.ScaleFit"=w240) -> ()  [unwired: 2 in, 2 out]
            n223 = Greater?(x=w234, y=u8 1) -> (0:w236:bool)
            n224 = Select(t=i8 0 ("cas vrai"), s=w236, f=i8 2 ("cas faux")) -> (s? t:f=w237:i8)
            n225 = property on="Graphe" class="GraphXY (strict)"("XScale.ScaleFit"=w237) -> ()  [unwired: 2 in, 2 out]
          }
        }
        n226 = case shown="Vrai" w228 {
          tunnel: [_ w229] -> w215
          frame False {
          }
          frame True {
            n227 = local read "Tableau de chaînes"() -> (w229:string[])
          }
        }
        n228 = local read "Curseur"() -> (w218:u16)
        n229 = property on="Curseur" class="MDér (strict)"("Strings []"=w215) -> ()  [unwired: 2 in, 2 out]
        n230 = Index Array(array=w215, index=w218) -> (element=w217:string)
        n231 = Search 1D Array(1D array=w215, element=w217) -> (index of element=w224:i32)  [unwired: 1 in]
        n232 = property on="Graphe" class="GraphXY (strict)"("Curseur actif"=u32 0) -> (error out=w226:errorcluster)  [unwired: 2 in, 1 out]
        n233 = property on="Graphe" class="GraphXY (strict)"(error in=w226, "Cursor.CursorMode"=u32 1 ("Curseur.Mode du curseur")) -> (error out=w227:errorcluster)  [unwired: 1 in, 1 out]
        n234 = property on="Graphe" class="GraphXY (strict)"(error in=w227, "Curseur.Tracé du curseur"=w224) -> (error out=w219:errorcluster)  [unwired: 1 in, 1 out]
        n235 = property on="Graphe" class="GraphXY (strict)"(error in=w219) -> (error out=w220:errorcluster, "Cursor.Cursor X"=w223:dbl)  [unwired: 1 in, 1 out]
        n236 = To Time Stamp(1:w223) -> (0:w222:timestamp)
        n237 = local write "X"(w222) -> ()
        n238 = property on="Graphe" class="GraphXY (strict)"(error in=w220) -> ("Cursor.Cursor Y"=w221:dbl)  [unwired: 1 in, 2 out]
        n239 = local write "Y"(w221) -> ()
      }
      event "Quitter graphe": Value Change {
        n240 = event-data() -> ("NewVal"=w241:bool)  [unwired: 1 in, 5 out]
        n241 = invoke on="Tableau de chaînes" class="Tabl (strict)" method="RétablirValParDéfaut"() -> ()  [unwired: 3 in, 3 out]
      }
      event "Bouton Aide": Value Change {
        n242 = event-data() -> ()  [unwired: 1 in, 6 out]
        n243 = call <vilib>:"Application Directory.vi"() -> ("Application Directory"=w243:path)
        n244 = Build Path(base path=w243, name or relative path="Logiciel GRAPHE_Instruction.pdf" ("standard input")) -> (appended path=w242:path)
        n245 = call "Open PDF.vi"("Path"=w242) -> ()  [unwired: 5 in, 2 out]
      }
    }
  }
  n246 = property on="Mini" class="NumNb (strict)"("DisabledEnum"=w18) -> ()  [unwired: 2 in, 2 out]
  n247 = property on="Maxi" class="NumNb (strict)"("DisabledEnum"=w18) -> ()  [unwired: 2 in, 2 out]
  n248 = local write "Echelle Y"(w18) -> ()
  n249 = local write "X"(timestamp(0 s since 1904-01-01) ("X")) -> ()
  n250 = for {
    tunnel: "Tableau de chaînes" -> [w248] mode=indexing
    tunnel: [w245] -> w1
    i -> [w251]
    n251 = property on="Graphe" class="GraphXY (strict)"("LegAutosize"=TRUE ("Légende:Redimensionnement automatique")) -> (error out=w246:errorcluster)  [unwired: 2 in, 1 out]
    n252 = property on="Graphe" class="GraphXY (strict)"(error in=w246, "Active Plot"=w251) -> (error out=w252:errorcluster)  [unwired: 1 in, 1 out]
    n253 = property on="Graphe" class="GraphXY (strict)"(error in=w252, "Plot.Visible?"=TRUE ("Tracé.Visible")) -> (error out=w249:errorcluster)  [unwired: 1 in, 1 out]
    n254 = property on="Graphe" class="GraphXY (strict)"(error in=w249, "Plot.Plot Name"=w248) -> (error out=w245:errorcluster)  [unwired: 1 in, 1 out]
  }
  n255 = property on="Active maths" class="Bool (strict)"("Value"=FALSE ("Valeur (Signalisation)")) -> ()  [unwired: 2 in, 2 out]
  n256 = property on="Graphe" class="GraphXY (strict)"(error in=w1, "LegAutosize"=FALSE ("Légende:Redimensionnement automatique")) -> (error out=w3:errorcluster)  [unwired: 1 in, 1 out]
  n257 = property on="Graphe" class="GraphXY (strict)"(error in=w3, "LegPos"=T2 {"Left"=830, "Top"=34} ("Légende:Position")) -> (error out=w2:errorcluster)  [unwired: 1 in, 1 out]
  n258 = Array Size(array="Tableau de chaînes") -> (size(s)=w8:i32)
  "Nbre courbes" <- w8
  n259 = Greater?(x=w8, y=w9) -> (0:w10:bool)
  n260 = property on="Graphe" class="GraphXY (strict)"(error in=w2, "LegPlotMin"=w8) -> (error out=w11:errorcluster)  [unwired: 1 in, 1 out]
  n261 = Select(t=w9, s=w10, f=w8) -> (s? t:f=w7:i32)
  n262 = property on="Graphe" class="GraphXY (strict)"(error in=w11, "LegNumRows"=w7) -> ()  [unwired: 1 in, 2 out]
